vi "Download.vi"   [LabVIEW 2020, in "NI_SFTP.lvlib"]
doc: "Download one or more files. The instance VI determines how the file content is stored."
uses:
  <vilib>/net/SFTP/NI_SFTP.lvlib
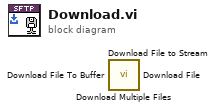
[diagram p0: block diagram]
diagram:
  n1 = call <vilib>:"Download Multiple Files.vi"() -> ()  [unwired: 10 in, 2 out]
  n2 = call <vilib>:"Download File to Stream.vi"() -> ()  [unwired: 9 in, 3 out]
  n3 = call <vilib>:"Download File To Buffer.vi"() -> ()  [unwired: 9 in, 3 out]
  n4 = call <vilib>:"Download File.vi"() -> ()  [unwired: 10 in, 2 out]
